vi "Counter to DAC.vi"() -> ()   [LabVIEW 2014]
uses:
  <vilib>/Platform/TimedLoop/XDataNode/XDataNode.xnode
  <vilib>/Platform/TimedLoop/XDataNode/nitl_modes.ctl
  <vilib>/Platform/TimedLoop/XDataNode/XDNodeRunTimeDep.lvlib
  <vilib>/Platform/TimedLoop/XDataNode/wakeup.ctl
  <vilib>/Platform/TimedLoop/XDataNode/timing_clust.ctl
  <vilib>/eio/EIONode/EIONode.xnode
  <vilib>/rvi/eio/common/nirviEmuTemplateMethod_errors.vi
  <vilib>/rvi/DataTransferAndStorage/Container/XNode/niFpgaContainer.xnode
  <vilib>/rvi/interface/RandomDataEmulation/nirviRandomDataFpgaReadWriteTemplate.vi
panel:
  in  "Scale 2":i16=100
  in  "Scale 1":i16=100
  in  "Offset 2":i16
  in  "Offset 1":i16
  in  "Counter ticks":u32=40000
  out "Ctr Elapsed":u32
  out "Ctr transfer":u32
  out "Ctr Overflow?":bool
  in  "Ctr FIFO":bool
  in  "Outputs\nDIO 12-15":bool[](array[boolean])=[FALSE, FALSE, FALSE, FALSE]
  out "Inputs\nDIO 8-11":bool[](array[boolean])=[TRUE, FALSE, FALSE, FALSE]
  out "Counts":u32[](array[numeric])
  out "loop elapsed":u16
  in  "Rate":u32=400 caption="Count(Ticks)"
  out "DAC 2":i16
  out "DAC 1":i16
  in  "Dac2 sub":bool[](array[boolean])=[FALSE, FALSE, FALSE, FALSE, FALSE, FALSE, FALSE, FALSE]
  in  "Dac2 add":bool[](array[boolean])=[TRUE, TRUE, TRUE, TRUE, TRUE, TRUE, TRUE, FALSE]
  in  "Dac1 sub":bool[](array[boolean])=[FALSE, FALSE, FALSE, FALSE, FALSE, FALSE, FALSE, FALSE]
  in  "Dac1 add":bool[](array[boolean])=[TRUE, TRUE, TRUE, TRUE, TRUE, TRUE, TRUE, FALSE]
  # "Counter FIFO"
  # "Hz to Volts"
  # "TTL I/O"
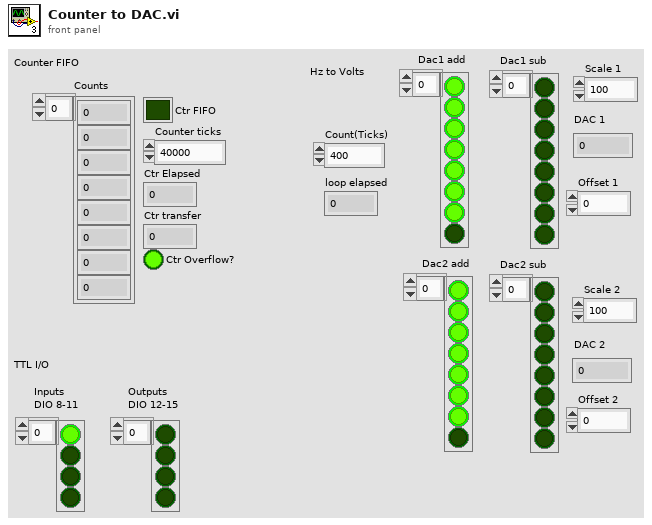
[diagram p1: front panel]
types:
  T1 = typedef "XDNodeRunTimeDep.lvlib/timing_clust.ctl" = cluster{"Expected End [f-1]":u64, "Actual End [f-1]":u64, "Finished Late? [f-1]":bool, "Expected End [i-1]":u64, "Actual End [i-1]":u64, "Finished Late? [i-1]":bool, "Expected Start [i]":u64, "Actual Start [i]":u64, "Expected Start [f]":u64, "Actual Start [f]":u64, "Source Name":string, "Structure Name":string, "Period":i64, "Deadline":i64, "Offset":i64, "Start":i64, "Priority":i32, "Timeout":i32, "Mode":T2, "Wakeup Reason":T3, "Error":errorcluster, "Source Type":string, "Secondary Source Type":string, "Global End Time":u64, "Global Start Time":u64, "Frame Duration":u64, "Iteration Duration":u64, "Assigned CPU":i32, "I/O Scan Engine Mode":u32}
  T2 = typedef "XDNodeRunTimeDep.lvlib/nitl_modes.ctl" = enum32{"No Change", "Process missed periods, maintain original phase", "Discard missed periods, maintain original phase", "Process missed periods, ignore original phase", "Discard missed periods, ignore original phase"}
  T3 = typedef "XDNodeRunTimeDep.lvlib/wakeup.ctl" = enum32{"Normal", "Aborted", "Asynchronous wakeup", "Timing source error", "Timed loop error", "Timeout"}
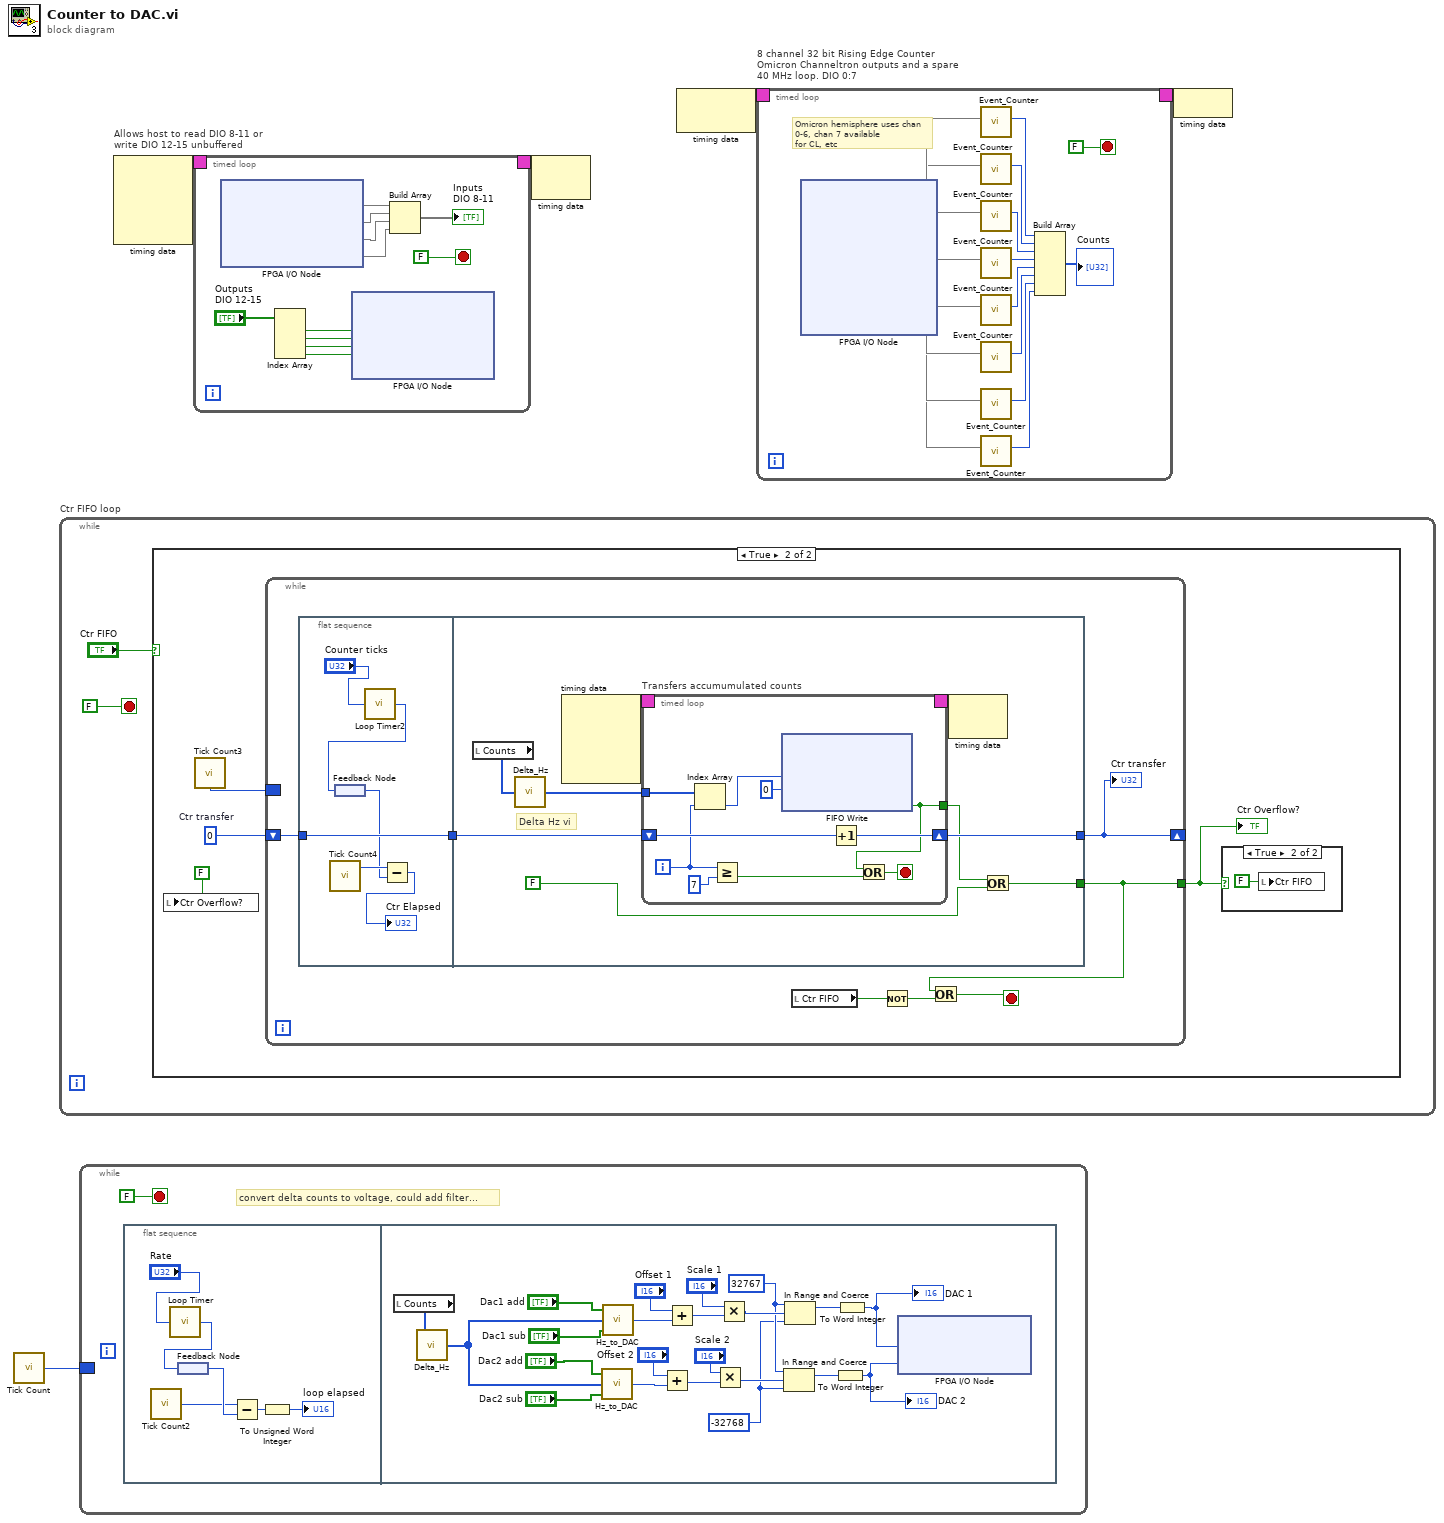
[diagram p0: block diagram]
diagram:
  n1 = call "Tick Count"() -> ("Tick Count(Ticks)"=w3:u32)
  n2 = while "Ctr FIFO loop" {
    stop <- FALSE stop-if-true
    n3 = case shown="True" "Ctr FIFO" {
      frame False {
      }
      frame True {
        w11 = u32 0  # Ctr transfer
        n4 = local write "Ctr Overflow?"(FALSE ("AI Buffer Overflow?")) -> ()
        n5 = call "Tick Count3"() -> ("Tick Count(Ticks)"=w8:u32)
        n6 = while {
          shift-right: [w17] -> _
          shift-left: w11 -> [w18]
          tunnel: [w15] -> w9
          border: w8 -> [_]
          stop <- w16 stop-if-true
          n7 = flat-sequence {
            tunnel: [w25] -> w19
            tunnel: w18 -> [w25]
            tunnel: w19 -> [w34]
            tunnel: [w33] -> w17
            tunnel: [w30] -> w15
            frame #0 {
              n8 = call "Tick Count4"() -> ("Tick Count(Ticks)"=w22:u32)
              n9 = feedback #1() -> (w21:u32)
              n10 = call "Loop Timer2"("Count(Ticks)"="Counter ticks") -> ("Tick Count(Ticks)"=w20:u32)
              n11 = feedback-in #1(w20) -> ()
              n12 = Subtract(x=w22, y=w21) -> (x-y=→"Ctr Elapsed":u32)
            }
            frame #1 {
              # "Delta Hz vi"
              n13 = local read "Counts"() -> (w32:u32[])
              n14 = call "Delta_Hz.vi"("Counts"=w32) -> ("Delta"=w31:i32[])
              n15 = node-c288() -> (w28:T1)  [unwired: 4 in]
              n16 = timed-loop "Transfers accumumulated counts" {
                timing: w28 -> [_]
                timing-out: [_] -> w27
                shift-right: [w43] -> w33
                shift-left: w34 -> [w44]
                tunnel: [w35] -> w26
                tunnel: w31 -> [w41]
                i -> [w39]
                stop <- w37 stop-if-true
                n17 = Index Array(array=w41, index=w39) -> (element=w40:i32)
                n18 = Greater Or Equal?(x=w39, y=7) -> (x >= y?=w36:bool)
                n19 = xnode ("FIFO Write")("Element"=w40, "Timeout"=0) -> ("Timed Out?"=w35:bool)  [unwired: 1 in, 1 out]
                n20 = Increment(x=w44) -> (x+1=w43:u32)
                n21 = Or(x=w35, y=w36) -> (x .or. y?=w37:bool)
              }
              n22 = node-c288(w27) -> ()  [unwired: 1 out]
              n23 = Or(x=w26, y=FALSE) -> (x .or. y?=w30:bool)
            }
          }
          n24 = local read "Ctr FIFO"() -> (w14:bool)
          n25 = Not(x=w14) -> (.not. x?=w13:bool)
          n26 = Or(x=w15, y=w13) -> (x .or. y?=w16:bool)
          "Ctr transfer" <- w17
        }
        "Ctr Overflow?" <- w9
        n27 = case shown="True" w9 {
          frame False {
          }
          frame True {
            n28 = local write "Ctr FIFO"(FALSE ("Ctr FIFO")) -> ()
          }
        }
      }
    }
  }
  n29 = while {
    border: w3 -> [_]
    stop <- FALSE stop-if-true
    # "convert delta counts to voltage, could add filter..."
    n30 = flat-sequence {
      frame #0 {
        n31 = call "Tick Count2"() -> ("Tick Count(Ticks)"=w52:u32)
        n32 = call "Loop Timer"("Count(Ticks)"="Rate") -> ("Tick Count(Ticks)"=w53:u32)
        n33 = feedback #2() -> (w55:u32)
        n34 = feedback-in #2(w53) -> ()
        n35 = Subtract(x=w52, y=w55) -> (x-y=w50:u32)
        n36 = To Unsigned Word Integer(number=w50) -> (unsigned 16bit integer=→"loop elapsed":u16)
      }
      frame #1 {
        w60 = -32768 ("lower limit")
        w61 = 32767 ("upper limit")
        n37 = local read "Counts"() -> (w76:u32[])
        n38 = call "Delta_Hz.vi"("Counts"=w76) -> ("Delta"=w77:i32[])
        n39 = call "Hz_to_DAC.vi"("Subtract"="Dac2 sub", "Delta"=w77, "Add"="Dac2 add") -> ("Output counts"=w68:i32)
        n40 = call "Hz_to_DAC.vi"("Subtract"="Dac1 sub", "Delta"=w77, "Add"="Dac1 add") -> ("Output counts"=w71:i32)
        n41 = Add(x="Offset 2", y=w68) -> (x+y=w64:i32)
        n42 = Add(x="Offset 1", y=w71) -> (x+y=w67:i32)
        n43 = Multiply(x="Scale 2", y=w64) -> (x*y=w62:i32)
        n44 = Multiply(x="Scale 1", y=w67) -> (x*y=w63:i32)
        n45 = In Range and Coerce(upper limit=w61, x=w62, lower limit=w60) -> (coerced(x)=w57:i32)  [unwired: 1 out]
        n46 = In Range and Coerce(upper limit=w61, x=w63, lower limit=w60) -> (coerced(x)=w59:i32)  [unwired: 1 out]
        n47 = To Word Integer(number=w57) -> (16bit integer=w56:i16)
        "DAC 2" <- w56
        n48 = To Word Integer(number=w59) -> (16bit integer=w58:i16)
        "DAC 1" <- w58
        n49 = xnode "FPGA I/O Node"("Connector0/AO0"=w58, "Connector0/AO1"=w56) -> ()  [unwired: 3 in, 3 out]
      }
    }
  }
  n50 = node-c288() -> (w2:T1)  [unwired: 4 in]
  n51 = timed-loop "Allows host to read DIO 8-11 or\nwrite DIO 12-15 unbuffered" {
    timing: w2 -> [_]
    timing-out: [_] -> w1
    stop <- FALSE stop-if-true
    n52 = xnode "FPGA I/O Node"() -> ("Connector0/DIO8"=w83, "Connector0/DIO9"=w85, "Connector0/DIO10"=w86, "Connector0/DIO11"=w87)  [unwired: 4 in, 4 out]
    n53 = Index Array(array="Outputs\nDIO 12-15") -> (element #1=w81:bool, element #2=w80:bool, element #3=w79:bool, element #4=w78:bool)  [unwired: 4 in]
    n54 = xnode "FPGA I/O Node"("Connector0/DIO12"=w81, "Connector0/DIO13"=w80, "Connector0/DIO14"=w79, "Connector0/DIO15"=w78) -> ()  [unwired: 4 in, 4 out]
    n55 = Build Array(w83, w85, w86, w87) -> (→"Inputs\nDIO 8-11":void[])
  }
  n56 = node-c288(w1) -> ()  [unwired: 1 out]
  n57 = node-c288() -> (w5:T1)  [unwired: 1 in]
  n58 = timed-loop "8 channel 32 bit Rising Edge Counter\nOmicron Channeltron outputs and a spare\n40 MHz loop. DIO 0:7" {
    timing: w5 -> [_]
    timing-out: [_] -> w4
    stop <- FALSE stop-if-true
    # "Omicron hemisphere uses chan 0-6, chan 7 available\nfor CL, etc"
    n59 = xnode "FPGA I/O Node"() -> ("Connector0/DIO0"=w107, "Connector0/DIO1"=w106, "Connector0/DIO2"=w105, "Connector0/DIO3"=w104, "Connector0/DIO4"=w103, "Connector0/DIO5"=w102, "Connector0/DIO6"=w101, "Connector0/DIO7"=w100)  [unwired: 8 in, 8 out]
    n60 = call "Event_Counter.vi"("input"=w107) -> ("Counts"=w99:u32)  [unwired: 10 in]
    n61 = call "Event_Counter.vi"("input"=w106) -> ("Counts"=w98:u32)  [unwired: 10 in]
    n62 = call "Event_Counter.vi"("input"=w105) -> ("Counts"=w97:u32)  [unwired: 10 in]
    n63 = call "Event_Counter.vi"("input"=w104) -> ("Counts"=w96:u32)  [unwired: 10 in]
    n64 = call "Event_Counter.vi"("input"=w103) -> ("Counts"=w95:u32)  [unwired: 10 in]
    n65 = call "Event_Counter.vi"("input"=w102) -> ("Counts"=w94:u32)  [unwired: 10 in]
    n66 = call "Event_Counter.vi"("input"=w101) -> ("Counts"=w93:u32)  [unwired: 10 in]
    n67 = call "Event_Counter.vi"("input"=w100) -> ("Counts"=w92:u32)  [unwired: 10 in]
    n68 = Build Array(w99, w98, w97, w96, w95, w94, w93, w92) -> (→"Counts":u32[])
  }
  n69 = node-c288(w4) -> ()
